vi "New Drive Train Status.vi"(8 "error in (no error)":errorcluster, 10 "Drive Train Status":T1 {"Right Power Setpoint" min=-1.0 max=1.0 step=0.1 scale=-1.0..1.0; "Left Power Setpoint" min=-1.0 max=1.0 step=0.1 scale=-1.0..1.0; "Right Power" min=-1.0 max=1.0 step=0.1 scale=-1.0..1.0; "Left Power" min=-1.0 max=1.0 step=0.1 scale=-1.0..1.0}, 11 "Drive by Power in":refnum<class "Drive by Power.lvclass">) -> (0 "error out":errorcluster, 3 "Drive by Power out":refnum<class "Drive by Power.lvclass">)   [LabVIEW 2014, in "Logical Systems.lvlib" / "Drive Train.lvlib" / "Drive by Power.lvlib" / "Drive by Power.lvclass"]
uses:
  Drive by Power.lvclass
  Drive Train Class/Drive Train Status.ctl
  Drive Train Command/Drive Train Command Class/Drive Train Command.lvclass
  Drive Train Class/Drive Train.lvclass
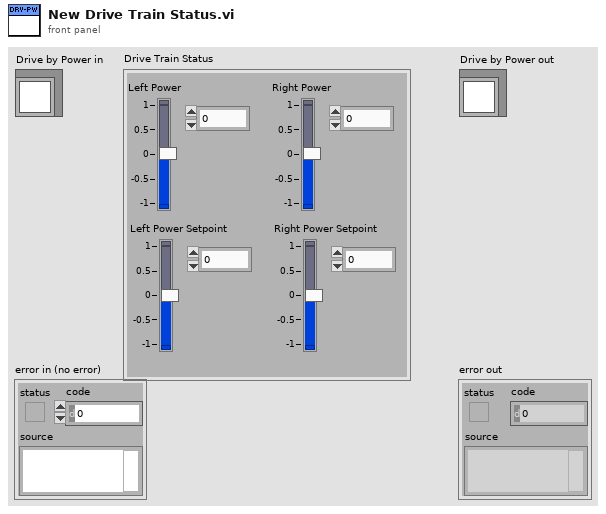
[diagram p1: front panel]
types:
  T1 = typedef "Logical Systems.lvlib/Drive Train.lvlib/Drive Train.lvclass/Drive Train Status.ctl" = cluster{"Left Power":dbl, "Right Power":dbl, "Left Power Setpoint":dbl, "Right Power Setpoint":dbl}
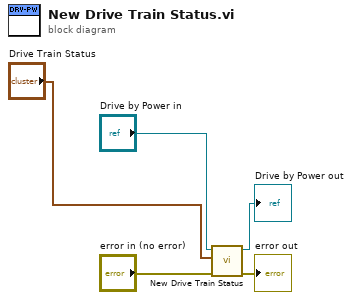
[diagram p0: block diagram]
diagram:
  n1 = call-parent "New Drive Train Status.vi"("error in (no error)"="error in (no error)", "Drive Train Status"="Drive Train Status", "Drive Train Command in"="Drive by Power in") -> ("error out"=→"error out":errorcluster, "Drive Train Command out"=→"Drive by Power out":refnum<class "Drive by Power.lvclass">)  [unwired: 7 in]
